vi "balance.vi"(0 "Joystick X":dbl, 1 "Joystick Y":dbl) -> (2 "Drive Type":bool, 3 "left":dbl, 4 "right":dbl)   [LabVIEW 2011]
doc: "We call this VLAD (Very Literal Assisted Driving). VLAD balances bridges for us. VLAD will let the driver keep control, until is senses the bridge tip, at which point, it will take over the robot. VLAD uses a gyro and an accelerometer to make sure the bridge is balanced and will correct for an un-balanced bridge."
uses:
  fg_typedef.ctl
  DB DataType Custom.ctl
  ADXL345 I2C Axis.ctl
  <vilib>/addons/control/pid/pid.llb/PID Control Input Filter (DBL).vi
  <vilib>/addons/control/pid/pid.llb/PID (DBL).vi
  <vilib>/addons/control/pid/NI_PID_pid.lvlib
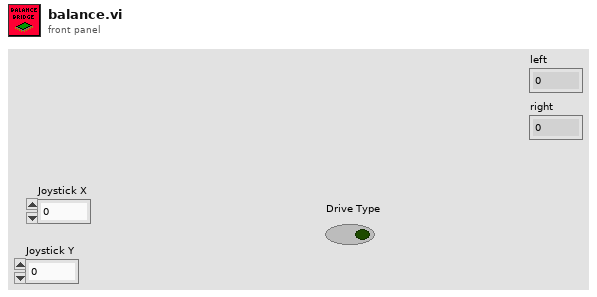
[diagram p1: front panel]
types:
  T1 = typedef "DB DataType Custom.ctl" = enum16{"VLAD Balanced", "Turret Safety", "Turret Limit"}
  T2 = typedef "fg_typedef.ctl" = enum16{"Get", "Set"}
  T3 = typedef "WPI_I2CDevRef.ctl" = cluster{"DevStatus":errorcluster, "Digital Module":T4, "Device Address":u8}
  T4 = typedef "FPGA_TypedefDigitalModule.ctl" = enum16{"Digital Module 1", "Digital Module 2"}
  T5 = typedef "WPI_GyroDevRef.ctl" = cluster{"DevStatus":errorcluster, "Analog Module":T6, "Analog Channel":T7, "Offset":dbl, "Gain (VoltsPerDegree/Second)":dbl}
  T6 = typedef "FPGA_TypedefAnalogModule.ctl" = enum16{"Analog Module 1", "Analog Module 2"}
  T7 = typedef "FPGA_AIChannel.ctl" = enum8{"AI 1", "AI 2", "AI 3", "AI 4", "AI 5", "AI 6", "AI 7", "AI 8", "Invalid"}
  T8 = typedef "WPI_EncoderDevRef.ctl" = cluster{"DevStatus":errorcluster, "EncoderIndex":T9, "CounterIndex":T10, "DistancePerCount":dbl, "Decoding Type":T11}
  T9 = typedef "FPGA_EncoderIdx.ctl" = enum8{"Enc 0", "Enc 1", "Enc 2", "Enc 3", "Invalid"}
  T10 = typedef "FPGA_CounterCtrSystemIndex.ctl" = enum8{"Ctr 0", "Ctr 1", "Ctr 2", "Ctr 3", "Ctr 4", "Ctr 5", "Ctr 6", "Ctr 7", "Invalid"}
  T11 = typedef "WPI_EncoderType.ctl" = enum16{"1x", "2x", "4x"}
  T12 = cluster{"proportional gain (Kc)":dbl, "integral time (Ti, min)":dbl, "derivative time (Td, min)":dbl}
  T13 = typedef "ADXL345 I2C Axis.ctl" = u8
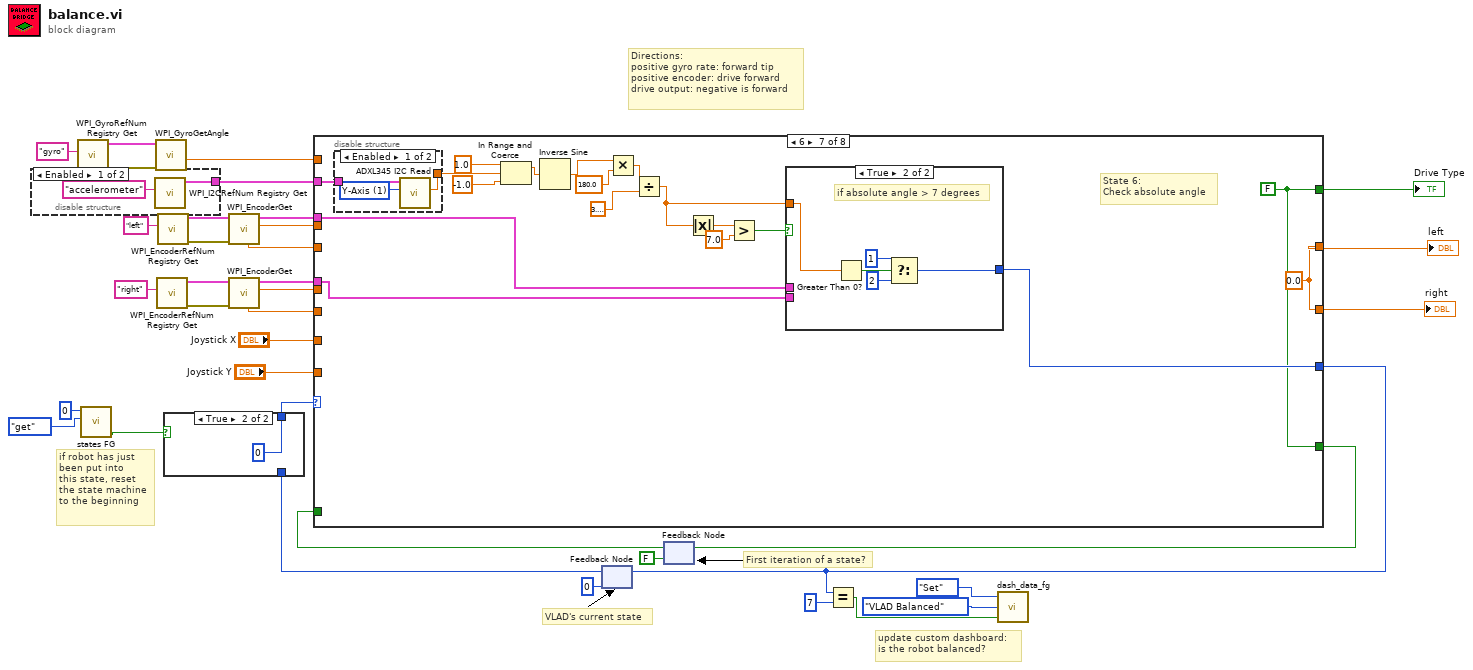
[diagram p0: block diagram]
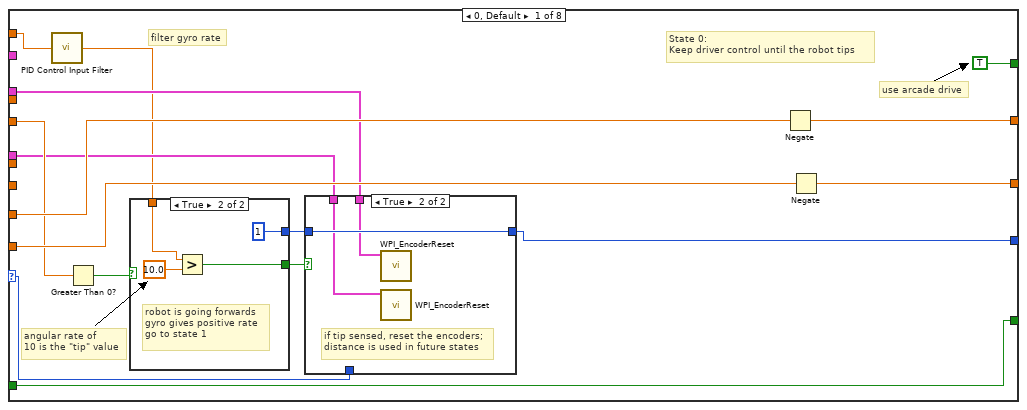
[diagram p4: hidden frame]
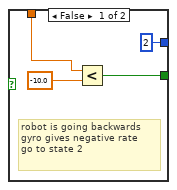
[diagram p6: hidden frame]
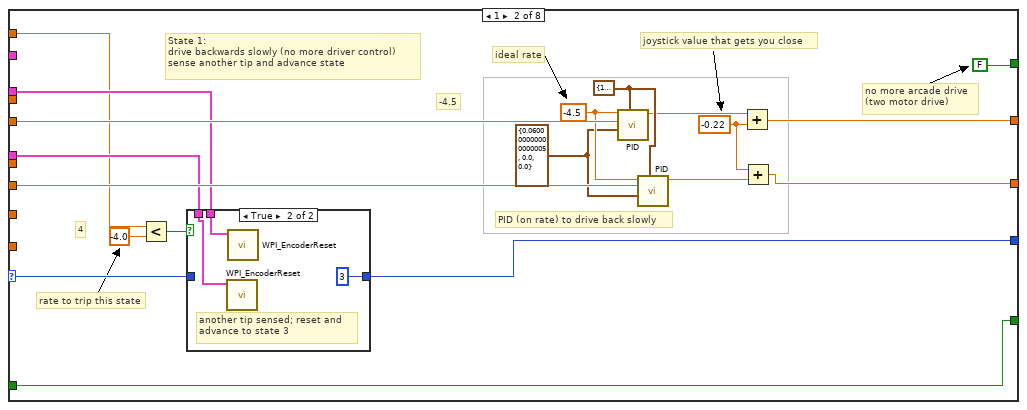
[diagram p7: hidden frame]
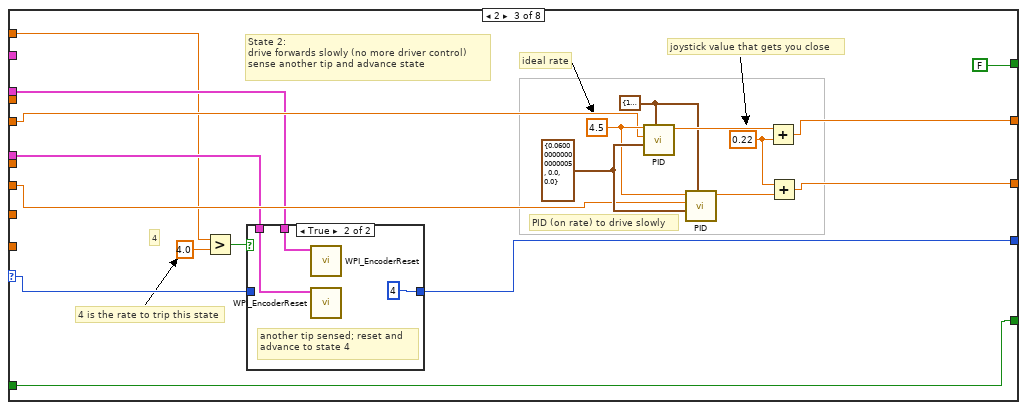
[diagram p9: hidden frame]
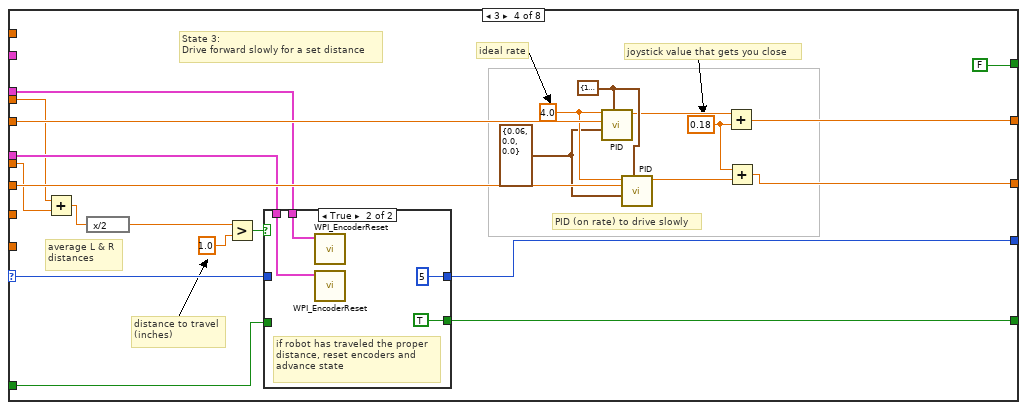
[diagram p11: hidden frame]
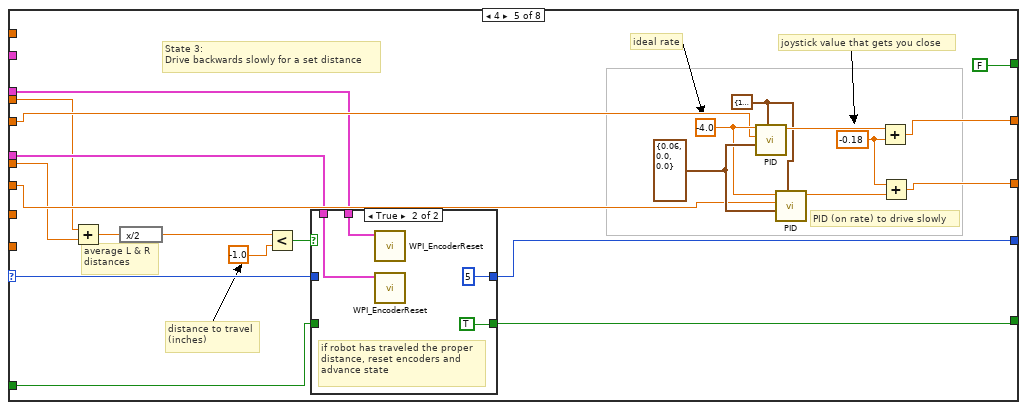
[diagram p13: hidden frame]
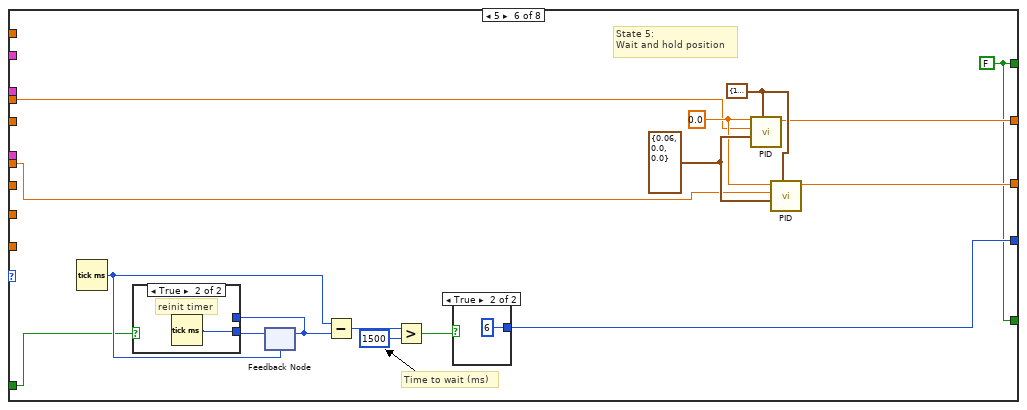
[diagram p15: hidden frame]
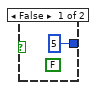
[diagram p16: hidden frame]
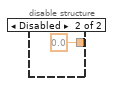
[diagram p18: hidden frame]
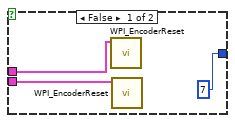
[diagram p19: hidden frame]
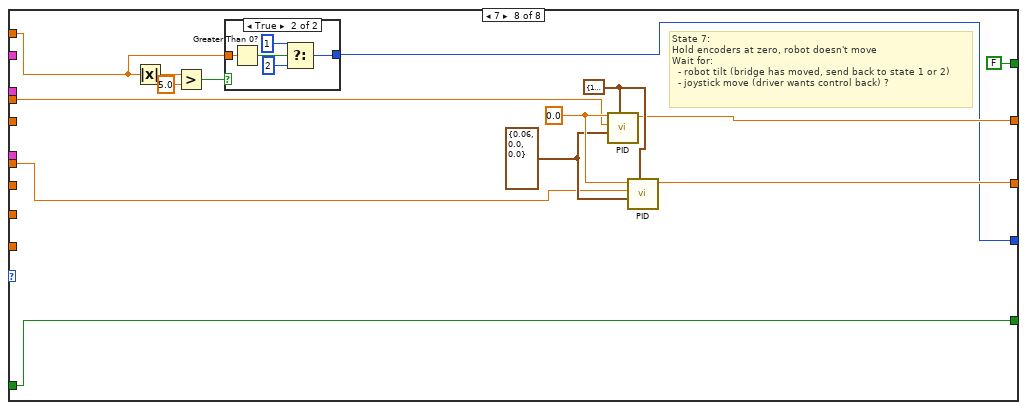
[diagram p20: hidden frame]
diagram:
  # "if robot has just \nbeen put into\nthis state, reset\nthe state machine\nto the beginning"
  # "update custom dashboard:\nis the robot balanced?"
  # "First iteration of a state?"
  # "Directions:\npositive gyro rate: forward tip\npositive encoder: drive forward\ndrive output: negative is forward"
  # "VLAD's current state"
  n1 = disable-structure shown="Enabled" {
    disable-tunnel: [w37 _] -> w16
    frame Enabled {
      n2 = call <vilib>:"WPI_I2CRefNum Registry Get.vi"("refnum name"="accelerometer") -> ("I2CDevRef"=w37:T3)  [unwired: 9 in, 1 out]
    }
    frame Disabled {
    }
  }
  n3 = call <vilib>:"WPI_GyroRefNum Registry Get.vi"("refnum name"="gyro") -> ("error out"=w23:errorcluster, "GyroDevRef"=w24:T5)  [unwired: 9 in]
  n4 = call "states FG.vi"("menu (get)"=enum16{"set", "get"}."get", "Loop ID"=0) -> ("first call?"=w8:bool)  [unwired: 6 in, 3 out]
  n5 = call <vilib>:"WPI_GyroGetAngle.vi"("error in (no error)"=w23, "GyroDevRef"=w24) -> ("Angular Rate"=w15:dbl)  [unwired: 6 in, 3 out]
  n6 = call <vilib>:"WPI_EncoderRefNum Registry Get.vi"("refnum name"="right") -> ("error out"=w31:errorcluster, "EncoderDevRef"=w33:T8)  [unwired: 9 in]
  n7 = call <vilib>:"WPI_EncoderRefNum Registry Get.vi"("refnum name"="left") -> ("error out"=w32:errorcluster, "EncoderDevRef"=w34:T8)  [unwired: 9 in]
  n8 = call <vilib>:"WPI_EncoderGet.vi"("error in (no error)"=w32, "EncoderDevRef"=w34) -> ("Distance"=w11:dbl, "EncoderDevRef"=w27:T8, "Rate"=w12:dbl)  [unwired: 4 in, 3 out]
  n9 = call <vilib>:"WPI_EncoderGet.vi"("error in (no error)"=w31, "EncoderDevRef"=w33) -> ("Distance"=w13:dbl, "EncoderDevRef"=w26:T8, "Rate"=w14:dbl)  [unwired: 4 in, 3 out]
  n10 = feedback #1(0) -> (w29:i32)
  n11 = case shown="True" w8 {
    tunnel: w29 -> [w39 _]
    tunnel: [w39 0] -> w28
    frame False {
    }
    frame True {
    }
  }
  n12 = feedback #2(FALSE) -> (w17:bool)
  n13 = case shown="6" w28 {
    selector: w28 -> [w49 w76 w99 w126 w155 _ _ _]
    tunnel: [w46 w75 w98 w125 w154 w181 w207 w223] -> w5
    tunnel: w12 -> [w53 w85 w103 w135 w159 _ _ _]
    tunnel: w14 -> [_ w84 w102 w134 w158 _ _ _]
    tunnel: [w41 w77 w101 w127 w157 w177 w203 w230] -> w10
    tunnel: [w42 w78 w100 w128 w156 w176 w203 w231] -> w9
    tunnel: w11 -> [_ _ _ w118 w147 w175 _ w233]
    tunnel: w13 -> [_ _ _ w117 w146 w174 _ w232]
    tunnel: w27 -> [w48 w74 w97 w124 w153 _ w205 _]
    tunnel: w26 -> [w47 w73 w96 w123 w152 _ w204 _]
    tunnel: w15 -> [w44 w71 w94 _ _ _ _ w224]
    tunnel: "Joystick X" -> [w56 _ _ _ _ _ _ _]
    tunnel: "Joystick Y" -> [w55 _ _ _ _ _ _ _]
    tunnel: [TRUE FALSE FALSE FALSE FALSE w173 w202 FALSE] -> w20
    tunnel: [w45 w70 w92 w116 w144 w173 w202 w228] -> w18
    tunnel: w17 -> [w45 w70 w92 w115 w145 w185 _ w228]
    tunnel: w16 -> [_ _ _ _ _ _ w206 _]
    frame 0, Default {
      # "use arcade drive"
      # "angular rate of\n10 is the \"tip\" value"
      # "filter gyro rate"
      # "State 0:\nKeep driver control until the robot tips"
      n14 = call-poly <vilib>:"PID Control Input Filter.vi"("input"=w44) -> ("output"=w43:dbl)  [unwired: 4 in]
      n15 = Greater Than 0?(x=w53) -> (x > 0?=w52:bool)
      n16 = case shown="True" w52 {
        tunnel: w43 -> [w64 w67]
        tunnel: [w62 w66] -> w51
        tunnel: [2 1] -> w50
        frame False {
          # "robot is going backwards\ngyro gives negative rate\ngo to state 2"
          n17 = Less?(x=w64, y=-10.0) -> (x < y?=w62:bool)
        }
        frame True {
          # "robot is going forwards\ngyro gives positive rate\ngo to state 1"
          n18 = Greater?(x=w67, y=10.0) -> (0:w66:bool)
        }
      }
      n19 = case shown="True" w51 {
        tunnel: w50 -> [_ w60]
        tunnel: w49 -> [w57 _]
        tunnel: w48 -> [_ w59]
        tunnel: w47 -> [_ w58]
        tunnel: [w57 w60] -> w46
        frame False {
          # "no tip sensed,\nhold this state"
        }
        frame True {
          # "if tip sensed, reset the encoders;\ndistance is used in future states"
          n20 = call <vilib>:"WPI_EncoderReset.vi"("EncoderDevRef"=w59) -> ()  [unwired: 9 in, 2 out]
          n21 = call <vilib>:"WPI_EncoderReset.vi"("EncoderDevRef"=w58) -> ()  [unwired: 9 in, 2 out]
        }
      }
      n22 = Negate(x=w56) -> (-x=w41:dbl)
      n23 = Negate(x=w55) -> (-x=w42:dbl)
    }
    frame 1 {
      w79 = -0.22 ("y")
      w82 = T12 {"proportional gain (Kc)"=0.060000000000000005, "integral time (Ti, min)"=0.0, "derivative time (Td, min)"=0.0} ("PID gains")
      w83 = -4.5
      w86 = cluster{"output high":dbl, "output low":dbl} {"output high"=1.0, "output low"=-1.0} ("output range")
      # "-4.5"
      # "4"
      # "joystick value that gets you close"
      # "ideal rate"
      # "rate to trip this state"
      # "PID (on rate) to drive back slowly"
      # "no more arcade drive\n(two motor drive)"
      # "State 1:\ndrive backwards slowly (no more driver control)\nsense another tip and advance state"
      n24 = Less?(x=w71, y=-4.0) -> (x < y?=w72:bool)
      n25 = case shown="True" w72 {
        tunnel: w76 -> [w88 _]
        tunnel: [w88 3] -> w75
        tunnel: w74 -> [_ w90]
        tunnel: w73 -> [_ w89]
        frame False {
          # "hold current state"
        }
        frame True {
          # "another tip sensed; reset and  \nadvance to state 3"
          n26 = call <vilib>:"WPI_EncoderReset.vi"("EncoderDevRef"=w89) -> ()  [unwired: 9 in, 2 out]
          n27 = call <vilib>:"WPI_EncoderReset.vi"("EncoderDevRef"=w90) -> ()  [unwired: 9 in, 2 out]
        }
      }
      n28 = call-poly <vilib>:"PID.vi"("output range"=w86, "PID gains"=w82, "process variable"=w85, "setpoint"=w83) -> ("output"=w81:dbl)  [unwired: 6 in, 1 out]
      n29 = call-poly <vilib>:"PID.vi"("output range"=w86, "PID gains"=w82, "process variable"=w84, "setpoint"=w83) -> ("output"=w80:dbl)  [unwired: 6 in, 1 out]
      n30 = Add(x=w81, y=w79) -> (x+y=w77:dbl)
      n31 = Add(x=w79, y=w80) -> (x+y=w78:dbl)
    }
    frame 2 {
      w109 = 0.22 ("y")
      w106 = T12 {"proportional gain (Kc)"=0.060000000000000005, "integral time (Ti, min)"=0.0, "derivative time (Td, min)"=0.0} ("PID gains")
      w105 = 4.5
      w104 = cluster{"output high":dbl, "output low":dbl} {"output high"=1.0, "output low"=-1.0} ("output range")
      # "4"
      # "joystick value that gets you close"
      # "ideal rate"
      # "PID (on rate) to drive slowly"
      # "4 is the rate to trip this state"
      # "State 2:\ndrive forwards slowly (no more driver control)\nsense another tip and advance state"
      n32 = Greater?(x=w94, y=4.0) -> (0:w93:bool)
      n33 = case shown="True" w93 {
        tunnel: w99 -> [w111 _]
        tunnel: [w111 4] -> w98
        tunnel: w97 -> [_ w113]
        tunnel: w96 -> [_ w112]
        frame False {
        }
        frame True {
          # "another tip sensed; reset and  \nadvance to state 4"
          n34 = call <vilib>:"WPI_EncoderReset.vi"("EncoderDevRef"=w113) -> ()  [unwired: 9 in, 2 out]
          n35 = call <vilib>:"WPI_EncoderReset.vi"("EncoderDevRef"=w112) -> ()  [unwired: 9 in, 2 out]
        }
      }
      n36 = call-poly <vilib>:"PID.vi"("output range"=w104, "PID gains"=w106, "process variable"=w103, "setpoint"=w105) -> ("output"=w107:dbl)  [unwired: 6 in, 1 out]
      n37 = call-poly <vilib>:"PID.vi"("output range"=w104, "PID gains"=w106, "process variable"=w102, "setpoint"=w105) -> ("output"=w108:dbl)  [unwired: 6 in, 1 out]
      n38 = Add(x=w107, y=w109) -> (x+y=w101:dbl)
      n39 = Add(x=w109, y=w108) -> (x+y=w100:dbl)
    }
    frame 3 {
      w129 = 0.18 ("y")
      w132 = T12 {"proportional gain (Kc)"=0.06, "integral time (Ti, min)"=0.0, "derivative time (Td, min)"=0.0} ("PID gains")
      w133 = 4.0
      w136 = cluster{"output high":dbl, "output low":dbl} {"output high"=1.0, "output low"=-1.0} ("output range")
      # "distance to travel\n(inches)"
      # "average L & R\ndistances"
      # "joystick value that gets you close"
      # "ideal rate"
      # "PID (on rate) to drive slowly"
      # "State 3:\nDrive forward slowly for a set distance"
      n40 = Add(x=w118, y=w117) -> (x+y=w119:dbl)
      n41 = expression code="x/2"(w119) -> (w121:dbl)
      n42 = Greater?(x=w121, y=1.0) -> (0:w120:bool)
      n43 = case shown="True" w120 {
        tunnel: w126 -> [w139 _]
        tunnel: [w139 5] -> w125
        tunnel: w124 -> [_ w142]
        tunnel: w123 -> [_ w141]
        tunnel: [w138 TRUE] -> w116
        tunnel: w115 -> [w138 _]
        frame False {
        }
        frame True {
          # "if robot has traveled the proper\ndistance, reset encoders and \nadvance state"
          n44 = call <vilib>:"WPI_EncoderReset.vi"("EncoderDevRef"=w142) -> ()  [unwired: 9 in, 2 out]
          n45 = call <vilib>:"WPI_EncoderReset.vi"("EncoderDevRef"=w141) -> ()  [unwired: 9 in, 2 out]
        }
      }
      n46 = call-poly <vilib>:"PID.vi"("output range"=w136, "PID gains"=w132, "process variable"=w135, "setpoint"=w133) -> ("output"=w131:dbl)  [unwired: 6 in, 1 out]
      n47 = call-poly <vilib>:"PID.vi"("output range"=w136, "PID gains"=w132, "process variable"=w134, "setpoint"=w133) -> ("output"=w130:dbl)  [unwired: 6 in, 1 out]
      n48 = Add(x=w131, y=w129) -> (x+y=w127:dbl)
      n49 = Add(x=w129, y=w130) -> (x+y=w128:dbl)
    }
    frame 4 {
      w165 = -0.18 ("y")
      w162 = T12 {"proportional gain (Kc)"=0.06, "integral time (Ti, min)"=0.0, "derivative time (Td, min)"=0.0} ("PID gains")
      w161 = -4.0
      w160 = cluster{"output high":dbl, "output low":dbl} {"output high"=1.0, "output low"=-1.0} ("output range")
      # "State 3:\nDrive backwards slowly for a set distance"
      # "average L & R\ndistances"
      # "distance to travel\n(inches)"
      # "joystick value that gets you close"
      # "ideal rate"
      # "PID (on rate) to drive slowly"
      n50 = Add(x=w147, y=w146) -> (x+y=w151:dbl)
      n51 = expression code="x/2"(w151) -> (w150:dbl)
      n52 = Less?(x=w150, y=-1.0) -> (x < y?=w148:bool)
      n53 = case shown="True" w148 {
        tunnel: w155 -> [w168 _]
        tunnel: [w168 5] -> w154
        tunnel: w153 -> [_ w171]
        tunnel: w152 -> [_ w170]
        tunnel: w145 -> [w167 _]
        tunnel: [w167 TRUE] -> w144
        frame False {
        }
        frame True {
          # "if robot has traveled the proper\ndistance, reset encoders and \nadvance state"
          n54 = call <vilib>:"WPI_EncoderReset.vi"("EncoderDevRef"=w171) -> ()  [unwired: 9 in, 2 out]
          n55 = call <vilib>:"WPI_EncoderReset.vi"("EncoderDevRef"=w170) -> ()  [unwired: 9 in, 2 out]
        }
      }
      n56 = call-poly <vilib>:"PID.vi"("output range"=w160, "PID gains"=w162, "process variable"=w159, "setpoint"=w161) -> ("output"=w163:dbl)  [unwired: 6 in, 1 out]
      n57 = call-poly <vilib>:"PID.vi"("output range"=w160, "PID gains"=w162, "process variable"=w158, "setpoint"=w161) -> ("output"=w164:dbl)  [unwired: 6 in, 1 out]
      n58 = Add(x=w163, y=w165) -> (x+y=w157:dbl)
      n59 = Add(x=w165, y=w164) -> (x+y=w156:dbl)
    }
    frame 5 {
      w180 = T12 {"proportional gain (Kc)"=0.06, "integral time (Ti, min)"=0.0, "derivative time (Td, min)"=0.0} ("PID gains")
      w179 = 0.0
      w178 = cluster{"output high":dbl, "output low":dbl} {"output high"=1.0, "output low"=-1.0} ("output range")
      w173 = FALSE
      # "Time to wait (ms)"
      # "State 5:\nWait and hold position"
      n60 = Tick Count (ms)() -> (millisecond timer value=w188:u32)
      n61 = feedback #3(w188) -> (w183:u32)
      n62 = case shown="True" w185 {
        tunnel: [w191 w192] -> w184
        tunnel: w183 -> [w191 _]
        frame False {
          # "not first call,\nkeep start\ntime"
        }
        frame True {
          # "reinit timer"
          n63 = Tick Count (ms)() -> (millisecond timer value=w192:u32)
        }
      }
      n64 = feedback-in #3(w184) -> ()
      n65 = Subtract(x=w188, y=w183) -> (x-y=w187:u32)
      n66 = Greater?(x=w187, y=u32 1500) -> (0:w182:bool)
      n67 = case shown="True" w182 {
        tunnel: [5 6] -> w181
        frame False {
          (unwired) FALSE
        }
        frame True {
        }
      }
      n68 = call-poly <vilib>:"PID.vi"("output range"=w178, "PID gains"=w180, "process variable"=w175, "setpoint"=w179) -> ("output"=w177:dbl)  [unwired: 6 in, 1 out]
      n69 = call-poly <vilib>:"PID.vi"("output range"=w178, "PID gains"=w180, "process variable"=w174, "setpoint"=w179) -> ("output"=w176:dbl)  [unwired: 6 in, 1 out]
    }
    frame 6 {
      w203 = 0.0
      w202 = FALSE
      # "State 6:\nCheck absolute angle"
      n70 = disable-structure shown="Enabled" {
        disable-tunnel: w206 -> [w212 _]
        disable-tunnel: [w211 0.0 ("Acceleration")] -> w194
        frame Enabled {
          w213 = T13 1 items=["X-Axis", "Y-Axis", "Z-Axis"] ("Axis")
          n71 = call "ADXL345 I2C Read.vi"("Axis"=w213, "I2CDevRef"=w212) -> ("Acceleration"=w211:dbl)  [unwired: 1 in, 8 out]
        }
        frame Disabled {
        }
      }
      n72 = In Range and Coerce(upper limit=1.0, x=w194, lower limit=-1.0) -> (coerced(x)=w197:dbl)  [unwired: 1 out]
      n73 = Inverse Sine(1:w197) -> (0:w198:dbl)
      n74 = Multiply(x=w198, y=180.0) -> (x*y=w199:dbl)
      n75 = Divide(x=w199, y=3.141592653589793) -> (x/y=w193:dbl)
      n76 = Absolute Value(x=w193) -> (abs(x)=w210:dbl)
      n77 = Greater?(x=w210, y=7.0) -> (0:w208:bool)
      n78 = case shown="True" w208 {
        tunnel: [7 w219] -> w207
        tunnel: w205 -> [w216 _]
        tunnel: w204 -> [w215 _]
        tunnel: w193 -> [_ w218]
        frame False {
          n79 = call <vilib>:"WPI_EncoderReset.vi"("EncoderDevRef"=w216) -> ()  [unwired: 9 in, 2 out]
          n80 = call <vilib>:"WPI_EncoderReset.vi"("EncoderDevRef"=w215) -> ()  [unwired: 9 in, 2 out]
        }
        frame True {
          # "if absolute angle > 7 degrees"
          n81 = Greater Than 0?(x=w218) -> (x > 0?=w220:bool)
          n82 = Select(t=1, s=w220, f=2) -> (s? t:f=w219:i32)
        }
      }
    }
    frame 7 {
      w234 = T12 {"proportional gain (Kc)"=0.06, "integral time (Ti, min)"=0.0, "derivative time (Td, min)"=0.0} ("PID gains")
      w235 = 0.0
      w236 = cluster{"output high":dbl, "output low":dbl} {"output high"=1.0, "output low"=-1.0} ("output range")
      # "State 7:\nHold encoders at zero, robot doesn't move\nWait for:\n  - robot tilt (bridge has moved, send back to state 1 or 2)\n  - joystick move (driver wants control back) ?"
      n83 = Absolute Value(x=w224) -> (abs(x)=w225:dbl)
      n84 = Greater?(x=w225, y=5.0) -> (0:w227:bool)
      n85 = case shown="True" w227 {
        tunnel: [7 w238] -> w223
        tunnel: w224 -> [_ w239]
        frame False {
        }
        frame True {
          n86 = Greater Than 0?(x=w239) -> (x > 0?=w240:bool)
          n87 = Select(t=1, s=w240, f=2) -> (s? t:f=w238:i32)
        }
      }
      n88 = call-poly <vilib>:"PID.vi"("output range"=w236, "PID gains"=w234, "process variable"=w233, "setpoint"=w235) -> ("output"=w230:dbl)  [unwired: 6 in, 1 out]
      n89 = call-poly <vilib>:"PID.vi"("output range"=w236, "PID gains"=w234, "process variable"=w232, "setpoint"=w235) -> ("output"=w231:dbl)  [unwired: 6 in, 1 out]
    }
  }
  "left" <- w10
  "right" <- w9
  "Drive Type" <- w20
  n90 = feedback-in #1(w5) -> ()
  n91 = feedback-in #2(w18) -> ()
  n92 = Equal?(x=w5, y=7) -> (x = y?=w3:bool)
  n93 = call "dash_data_fg.vi"("Input"=w3, "DB DataType"=DB_DataType_Custom."VLAD Balanced", "Menu (Get)"=fg_typedef."Set") -> ()  [unwired: 1 out]
